vi "DSC.Register.vi"(0 "HGF_DSCMonitor in":refnum<class "HGF_DSCMonitor.lvclass">, 2 "SV":refnum<k21>, 3 "HGF_NetworkVisitor":refnum<class "HGF_NetworkVisitor.lvclass">, 4 "Event Queue":refnum<queue>, 5 "error in (no error)":errorcluster, 7 "request changes (all changes)":u16(ring) items=["all changes", "value changes only"]) -> (14 "HGF_DSCMonitor out":refnum<class "HGF_DSCMonitor.lvclass">, 19 "error out":errorcluster)   [LabVIEW 2009]
uses:
  HGF_BaseClasses/HGF_NetworkVisitor/HGF_NetworkVisitor.lvclass
  HGF_DSCMonitor.lvclass
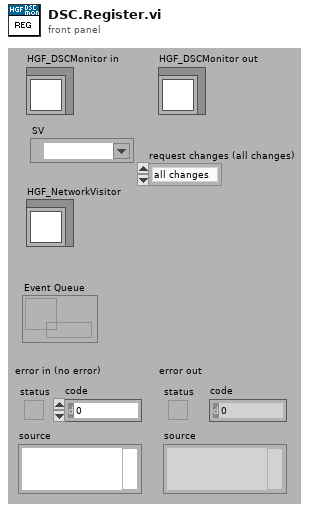
[diagram p1: front panel]
types:
  T1 = cluster{"Command":string, "SV":refnum<k21>, "HGF_NetworkVisitor":refnum<class "HGF_NetworkVisitor.lvclass">, "Event Queue":refnum<queue>, "request changes (all changes)":u16, "Switch":bool}
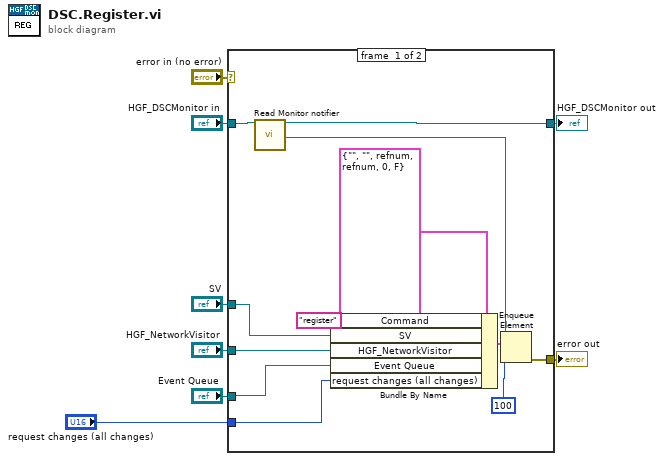
[diagram p0: block diagram]
diagram:
  n1 = case shown="No Error" "error in (no error)" {
    selector: "error in (no error)" -> [_ w22]
    tunnel: [w16 w22] -> w7
    tunnel: [w13 w21] -> w5
    tunnel: "HGF_DSCMonitor in" -> [w14 w21]
    tunnel: "SV" -> [w19 _]
    tunnel: "HGF_NetworkVisitor" -> [w18 _]
    tunnel: "Event Queue" -> [w17 _]
    tunnel: "request changes (all changes)" -> [w11 _]
    frame #0 {
      n2 = call "Read Monitor notifier.vi"("HGF_DSCMonitor.lvclass in"=w14) -> ("HGF_DSCMonitor.lvclass out"=w13:refnum<class "HGF_DSCMonitor.lvclass">, "Monitor Queue"=w10:refnum<queue>)  [unwired: 2 in, 15 out]
      n3 = Bundle By Name(cluster=T1 {"Command"="", "SV"="", "HGF_NetworkVisitor"=refnum, "Event Queue"=refnum, "request changes (all changes)"=0, "Switch"=FALSE} ("element"), "Command"="register", "SV"=w19, "HGF_NetworkVisitor"=w18, "Event Queue"=w17, "request changes (all changes)"=w11) -> (w12:T1)
      n4 = Enqueue Element(queue=w10, element=w12, timeout in ms (-1)=100) -> (error out=w16:errorcluster)  [unwired: 1 in, 2 out]
    }
    frame #1 {
    }
  }
  "error out" <- w7
  "HGF_DSCMonitor out" <- w5
